vi "Unregister MessageQ.vi"(8 "error in (no error)":errorcluster, 11 "Module in":refnum<class "Module.lvclass">) -> (0 "error out":errorcluster, 3 "Module out":refnum<class "Module.lvclass">)   [LabVIEW 2020, in "Volatus.lvlib" / "Module.lvclass"]
uses:
  Module.lvclass
  Module.lvclass/Module.ctl
  VolatusAPI/VolatusAPI.lvclass
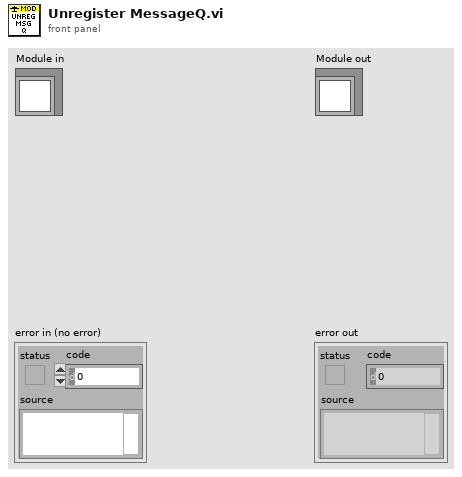
[diagram p1: front panel]
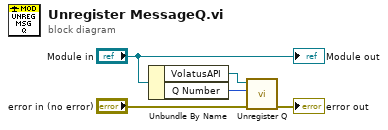
[diagram p0: block diagram]
diagram:
  n1 = Unbundle By Name("Module in") -> ("VolatusAPI"=w4:refnum<class "VolatusAPI.lvclass">, "Q Number"=w3:i32)
  n2 = call "Unregister Q.vi"("error in (no error)"="error in (no error)", "Q Number"=w3, "VolatusAPI in"=w4) -> ("error out"=→"error out":errorcluster)  [unwired: 7 in, 1 out]
  "Module out" <- "Module in"
